vi "Capture UI State SubVI.vi"(7 "Ctls Refs (All Ctls)":refnum<vi>[](array[refnum]), 8 "error in (no error)":errorcluster, 9 "ComboBox Text":string, 10 "Shift Pressed":bool, 11 "VI Ref In":refnum<vi>) -> (0 "error out":errorcluster)   [LabVIEW 2020, in "UIM.lvlib"]
uses:
  UIM.lvlib
  UIM.lvclass
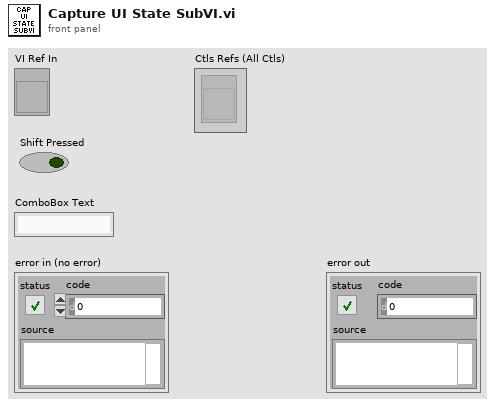
[diagram p1: front panel]
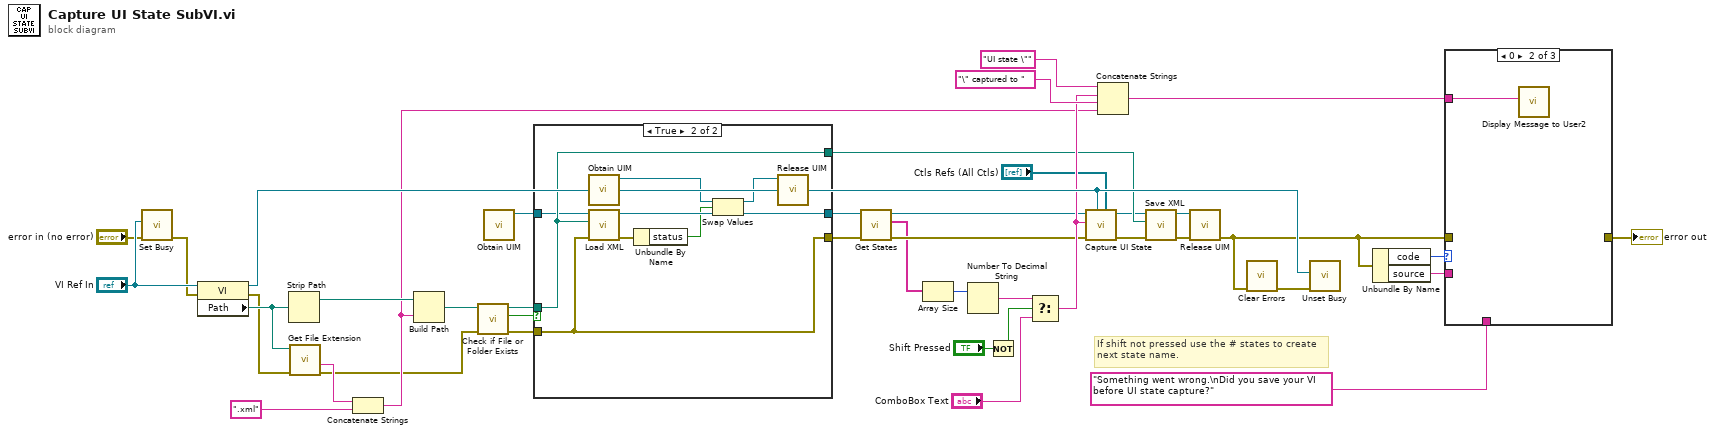
[diagram p0: block diagram]
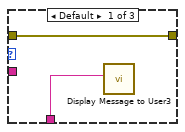
[diagram p2: hidden frame]
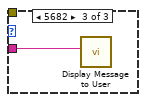
[diagram p3: hidden frame]
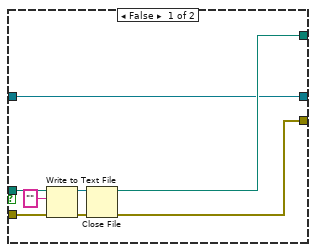
[diagram p4: hidden frame]
diagram:
  # "If shift not pressed use the # states to create\nnext state name."
  n1 = call <vilib>:"Set Busy.vi"("error in (no error)"="error in (no error)", "VI reference (current VI)"="VI Ref In") -> ("error out"=w16:errorcluster)  [unwired: 8 in, 1 out]
  n2 = property class="VI"(reference="VI Ref In", error in=w16) -> (reference out=w42:refnum<vi>, error out=w8:errorcluster, "Path"=w11:path)
  n3 = Strip Path(path=w11) -> (stripped path=w18:path)  [unwired: 1 out]
  n4 = call <vilib>:"Get File Extension.vi"("error in (no error)"=w8, "file"=w11) -> ("error out"=w7:errorcluster, "filename without extension"=w10:string)  [unwired: 5 in, 3 out]
  n5 = Concatenate Strings(w10, ".xml" ("string")) -> (w9:string)
  n6 = Build Path(base path=w18, name or relative path=w9) -> (appended path=w12:path)
  n7 = call <vilib>:"Check if File or Folder Exists.vi"("error in (no error)"=w7, "path"=w12) -> ("error out"=w22:errorcluster, "file or folder exists?"=w20:bool, "dup path"=w21:path)  [unwired: 7 in]
  n8 = call "Obtain UIM.vi"() -> ("UIM Handle"=w39:refnum<data-value>)  [unwired: 10 in, 1 out]
  n9 = case shown="True" w20 {
    tunnel: w21 -> [w50 w59]
    tunnel: w22 -> [w46 w51]
    tunnel: [w45 w59] -> w31
    tunnel: [w44 w51] -> w15
    tunnel: w39 -> [w43 w58]
    tunnel: [w43 w52] -> w40
    frame False {
      n10 = Write to Text File(file (use dialog)=w50, text="", error in=w46) -> (refnum out=w48:refnum<file>, error out=w47:errorcluster)  [unwired: 1 in, 1 out]
      n11 = Close File(refnum=w48, error in=w47) -> (path=w45:path, error out=w44:errorcluster)
    }
    frame True {
      n12 = call "Obtain UIM.vi"() -> ("UIM Handle"=w56:refnum<data-value>)  [unwired: 10 in, 1 out]
      n13 = call "Load XML.vi"("Error In"=w51, "XML File"=w59, "UIM In"=w58) -> ("Error Out"=w55:errorcluster, "UIM Out"=w57:refnum<data-value>)  [unwired: 7 in]
      n14 = Unbundle By Name(w55) -> ("status"=w54:bool)
      n15 = Swap Values(12:w56, 13:w54, 14:w57) -> (1:w53:refnum<data-value>, 3:w52:refnum<data-value>)
      n16 = call "Release UIM.vi"("UIM Handle"=w53) -> ()  [unwired: 10 in, 1 out]
    }
  }
  n17 = call "Get States.vi"("Error In"=w15, "UIM In"=w40) -> ("Error Out"=w29:errorcluster, "States"=w23:string[], "UIM Out"=w26:refnum<data-value>)  [unwired: 7 in]
  n18 = Array Size(array=w23) -> (size(s)=w24:i32)
  n19 = Number To Decimal String(number=w24) -> (decimal integer string=w25:string)  [unwired: 1 in]
  n20 = Not(x="Shift Pressed") -> (.not. x?=w13:bool)
  n21 = Select(t=w25, s=w13, f="ComboBox Text") -> (s? t:f=w36:string)
  n22 = call "Capture UI State.vi"("Ctls Refs (All Ctls)"="Ctls Refs (All Ctls)", "VI Ref (Calling VI)"=w42, "Error In"=w29, "State Name"=w36, "UIM In"=w26) -> ("Error Out"=w14:errorcluster, "UIM Out"=w30:refnum<data-value>)  [unwired: 5 in]
  n23 = Concatenate Strings("UI state \"", w36, "\" captured to " ("string"), w9) -> (w3:string)
  n24 = call "Save XML.vi"("Error In"=w14, "UIM XML Path"=w31, "UIM In"=w30) -> ("Error Out"=w33:errorcluster, "UIM Out"=w32:refnum<data-value>)  [unwired: 7 in]
  n25 = call "Release UIM.vi"("Error In"=w33, "UIM Handle"=w32) -> ("Error Out"=w4:errorcluster)  [unwired: 9 in]
  n26 = call <vilib>:"Clear Errors.vi"("error in (no error)"=w4) -> ("error out"=w38:errorcluster)  [unwired: 5 in, 1 out]
  n27 = call <vilib>:"Unset Busy.vi"("error in (no error)"=w38, "VI reference (current VI)"=w42) -> ()  [unwired: 9 in, 1 out]
  n28 = Unbundle By Name(w4) -> ("code"=w6:i32, "source"=w5:string)
  n29 = case shown="0" w6 {
    tunnel: [w61 _ _] -> w1
    tunnel: w4 -> [w61 _ _]
    tunnel: w5 -> [_ _ w63]
    tunnel: w3 -> [_ w62 _]
    tunnel: "Something went wrong.\nDid you save your VI before UI state capture?" ("string") -> [w60 _ _]
    frame Default {
      n30 = call "Display Message to User3"("Message"=w60) -> ()  [unwired: 9 in, 2 out]
    }
    frame 0 {
      n31 = call "Display Message to User2"("Message"=w62) -> ()  [unwired: 9 in, 2 out]
    }
    frame 5682 {
      n32 = call "Display Message to User"("Message"=w63) -> ()  [unwired: 9 in, 2 out]
    }
  }
  "error out" <- w1
